vi "core_singalling_write_error_handler.vi"(7 "modes (Sgnl)":T1(array[ring]), 8 "error in":errorcluster, 9 "control names":string[](array[string]), 10 "error?":bool[](array[boolean]), 11 "vi ref":refnum<vi>) -> (0 "error out":errorcluster, 3 "vi ref dup":refnum<vi>)   [LabVIEW 2015]
uses:
  polys/poly_ref_tools_eco_plus.vi
  <vilib>/Utility/error.llb/Clear Errors.vi
  <vilib>/Utility/Data Type/Get Type Information.vi
  <userlib>/_OpenG.lib/lvdata/lvdata.llb/Get Strings from Enum__ogtk.vi
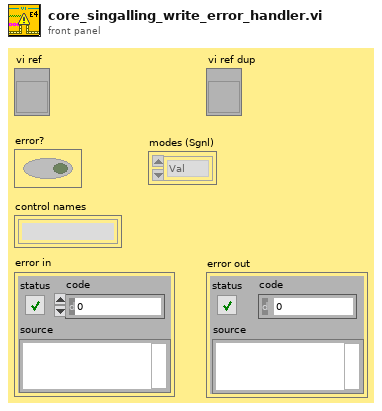
[diagram p1: front panel]
types:
  T1 = enum16{"Val", "Val(Sgnl)", "Val(Undo)", "Method"}[]
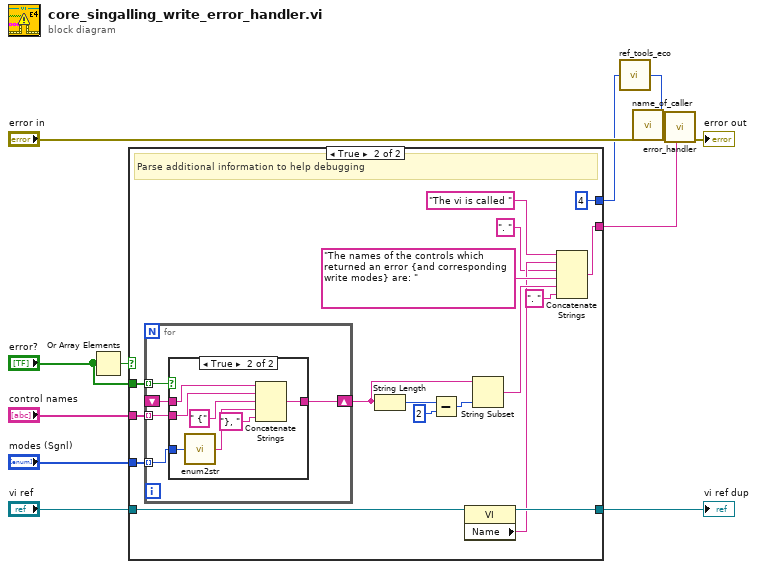
[diagram p0: block diagram]
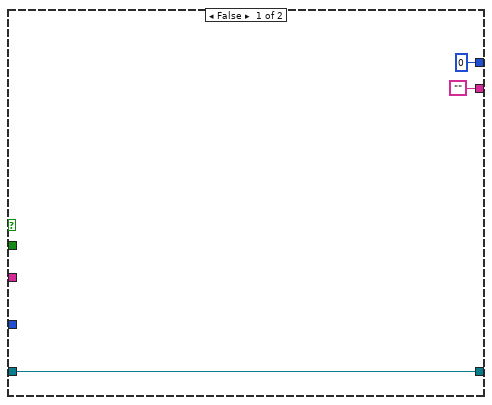
[diagram p2: hidden frame]
diagram:
  n1 = Or Array Elements(Boolean array="error?") -> (logical OR=w12:bool)
  n2 = case shown="True" w12 {
    tunnel: [0 4] -> w6
    tunnel: "error?" -> [_ w31]
    tunnel: "control names" -> [_ w30]
    tunnel: ["" w23] -> w11
    tunnel: "vi ref" -> [w13 w22]
    tunnel: [w13 w21] -> w9
    tunnel: "modes (Sgnl)" -> [_ w16]
    frame False {
    }
    frame True {
      # "Parse additional information to help debugging"
      n3 = for {
        tunnel: w31 -> [w35] mode=indexing
        tunnel: w30 -> [w37] mode=indexing
        shift-right: [w36] -> w27
        shift-left: _ -> [w34]
        tunnel: w16 -> [w33] mode=indexing
        n4 = case shown="True" w35 {
          tunnel: w37 -> [_ w45]
          tunnel: [w38 w44] -> w36
          tunnel: w34 -> [w38 w43]
          tunnel: w33 -> [_ w42]
          frame False {
          }
          frame True {
            n5 = call "enum2str.vi"("enum"=w42) -> ("element"=w40:string)
            n6 = Concatenate Strings(w43, w45, " {" ("string"), w40, "}, " ("string")) -> (w44:string)
          }
        }
      }
      n7 = String Length(string=w27) -> (length=w26:i32)
      n8 = Subtract(x=w26, y=2) -> (x-y=w24:i32)
      n9 = property class="VI"(reference=w22) -> (reference out=w21:refnum<vi>, "Name"=w19:string)  [unwired: 1 in, 1 out]
      n10 = String Subset(string=w27, length (rest)=w24) -> (substring=w28:string)  [unwired: 1 in]
      n11 = Concatenate Strings("The vi is called ", w19, ". " ("string"), "The names of the controls which returned an error {and corresponding write modes} are: ", w28, ". " ("string")) -> (w23:string)
    }
  }
  "vi ref dup" <- w9
  n12 = call-poly "ref_tools_eco.vi"("code (w/out eco)"=w6) -> ("code (+ eco)"=w5:i32)  [unwired: 4 in]
  n13 = call "name_of_caller.vi"() -> ("name of caller out"=w4:string)  [unwired: 4 in]
  n14 = call "error_handler.vi"("Additional info"=w11, "error in (no error)"="error in", "name of caller in (you)"=w4, "code (0 = no error)"=w5) -> ("error out"=→"error out":errorcluster)  [unwired: 6 in, 1 out]
